vi "主界面Z140.vi"() -> ()   [LabVIEW 2013]
uses:
  TCP/S7Ref.vi
panel:
  in  "复位":bool
  out "通讯状态":bool
  out "上序不合格":bool
  out "上序合格":bool
  out "本序不合格":bool
  out "本序合格":bool
  in  "停止":bool
  out "自动工步号":i32
  out "芯片ID":string
  out "压装工位操作状态":string
  in  "联线按钮":bool
  in  "选项卡控件":enum32{"自动界面", "手动界面", "参数"}(tab)
  out "胶塞在位":bool
  out "该型号检验辅具全在位，可以开始检验":bool
  out "辅具10":bool
  out "辅具9":bool
  out "辅具5":bool
  out "辅具4":bool
  out "辅具3":bool
  out "辅具2":bool
  out "辅具1":bool
  out "辅具6":bool
  in  "气缸进":bool
  in  "气缸退":bool
  out "联线状态":bool
  out "气压报警":bool
  in  "手动操作":bool
  in  "簇":T1
  out "员工ID":string
  out "员工姓名":string
  in  "型号选择":u16(ring)=1 items=["J709", "J706"]
  in  "参数加载":bool
  in  "产品ID":string
  # "芜湖机械转向器装配线"
  # "出厂检验台"
  # "Q14070机械转向器装配线"
  # "湖北唯思凌科装备制造有限公司 设计开发 (C)2015"
  # "检验前请检查辅具是否在位"
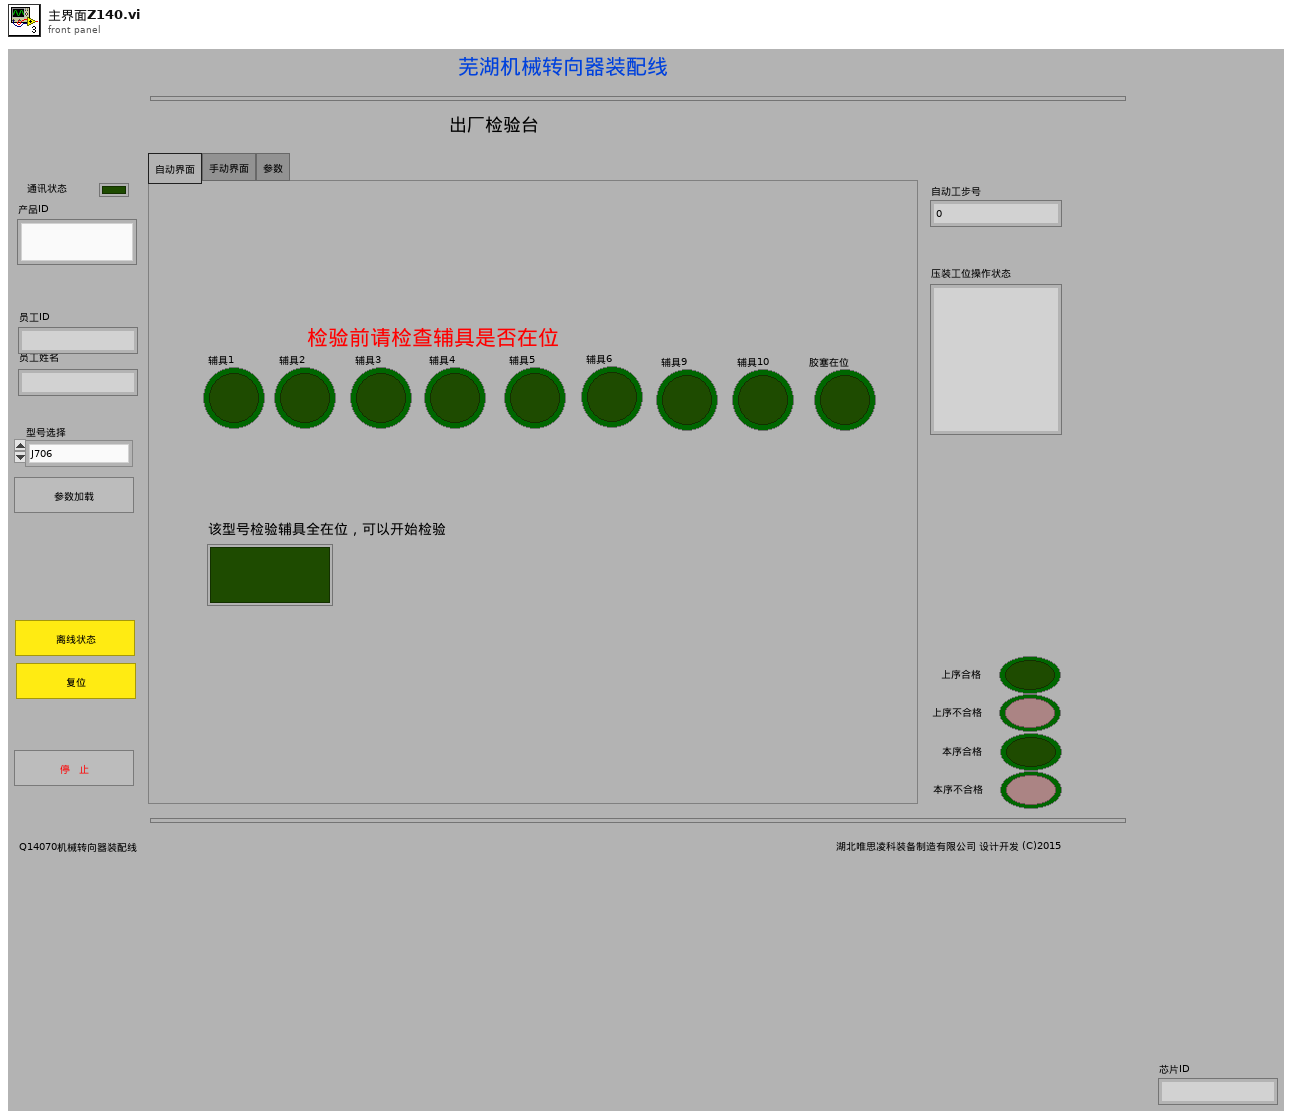
[diagram p1: front panel]
types:
  T1 = cluster{"布尔":bool, "布尔 2":bool, "布尔 3":bool, "布尔 4":bool, "布尔 5":bool, "布尔 6":bool, "布尔 7":bool, "布尔 8":bool, "布尔 9":bool}
  T2 = enum32{"Invalid", "Standard", "Closed", "Hidden", "Minimized", "Maximized"}
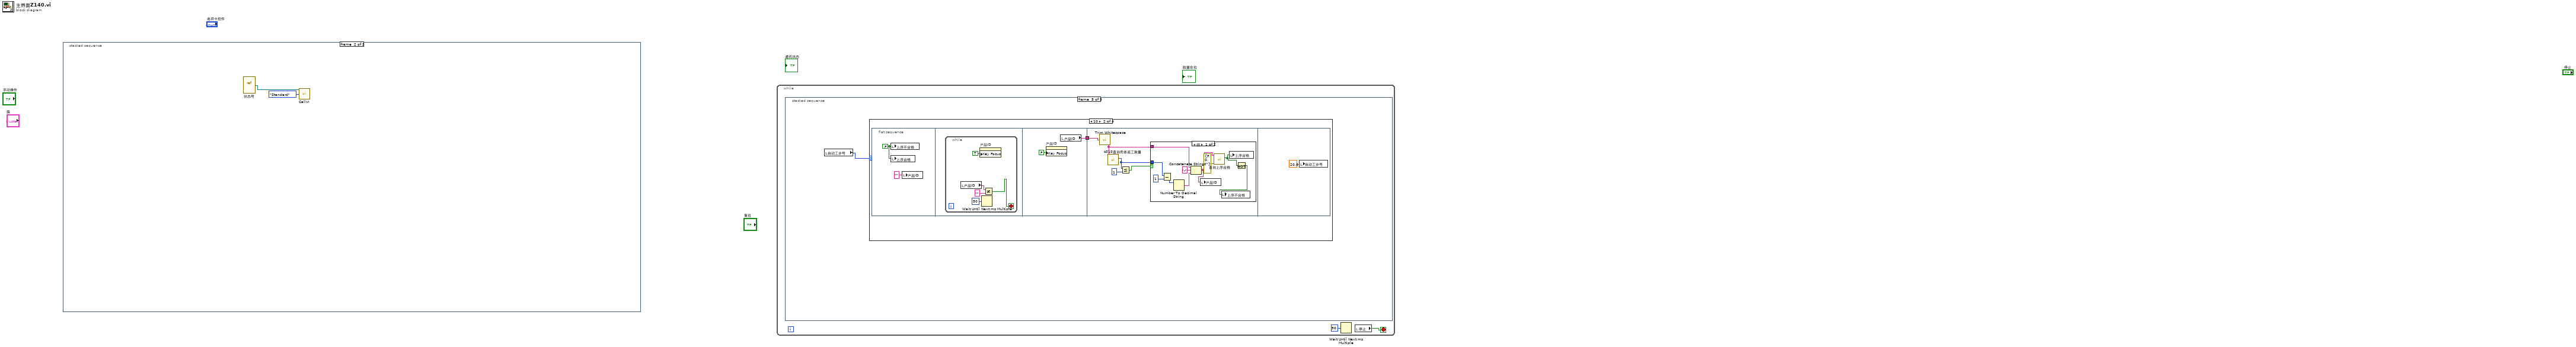
[diagram p0: block diagram]
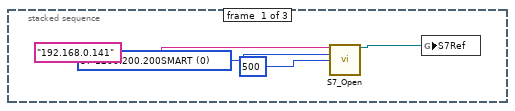
[diagram p2: hidden frame]
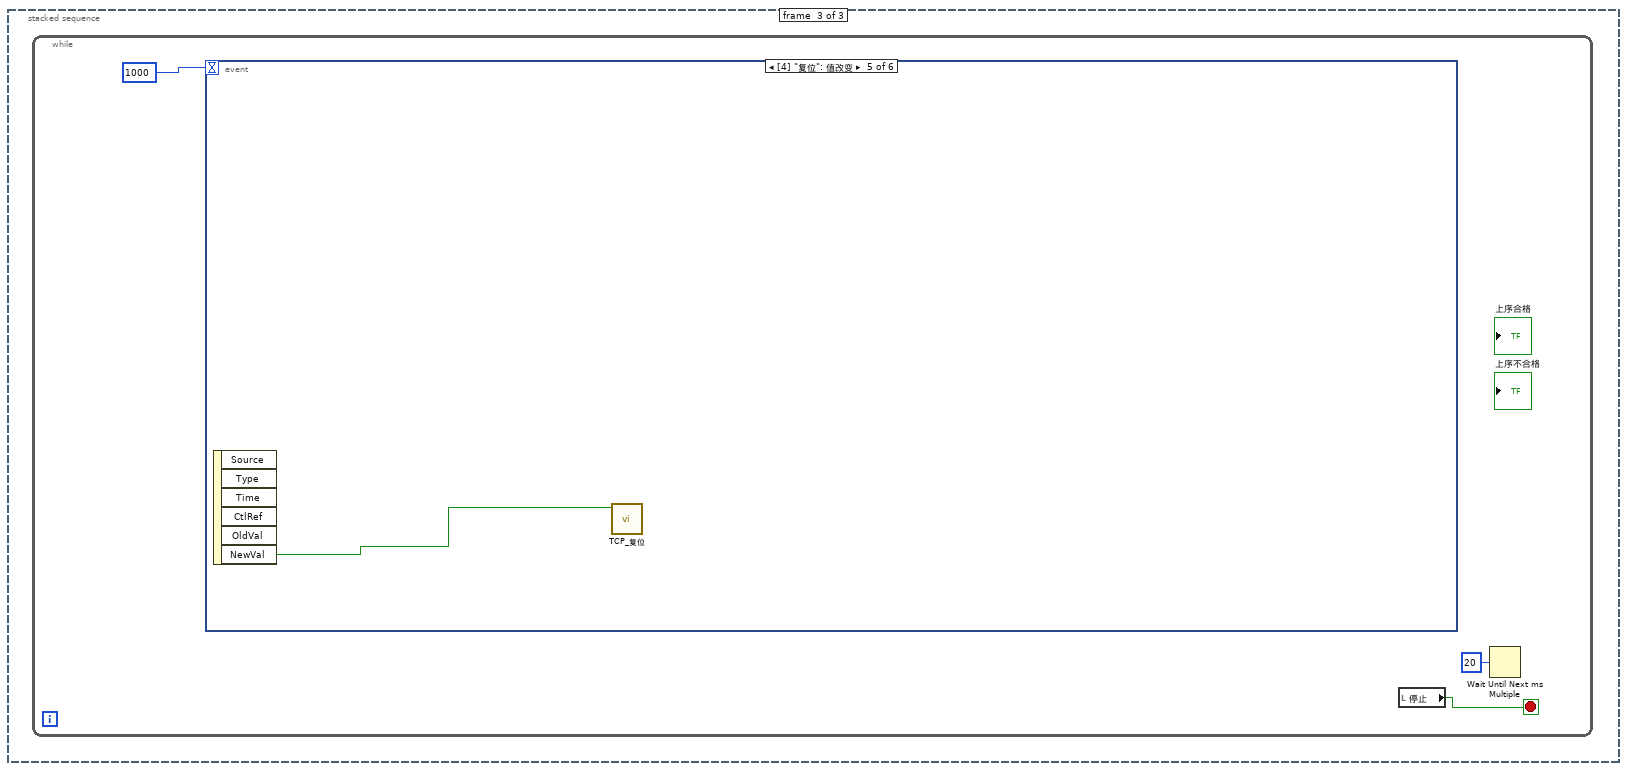
[diagram p3: hidden frame]
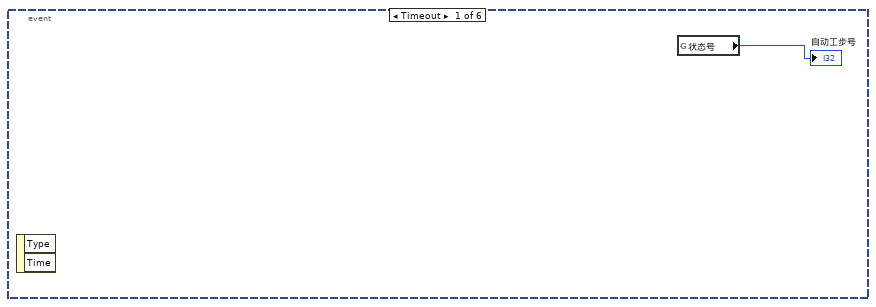
[diagram p4: hidden frame]
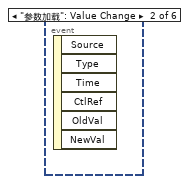
[diagram p5: hidden frame]
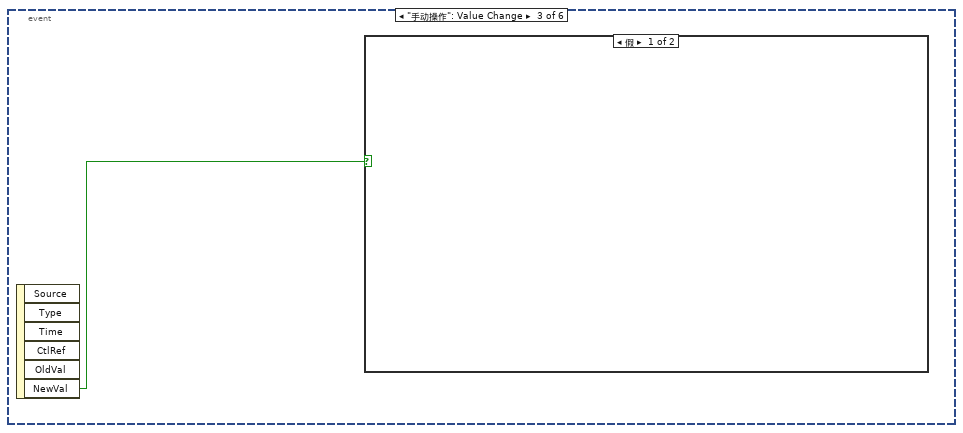
[diagram p6: hidden frame]
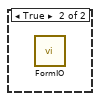
[diagram p7: hidden frame]
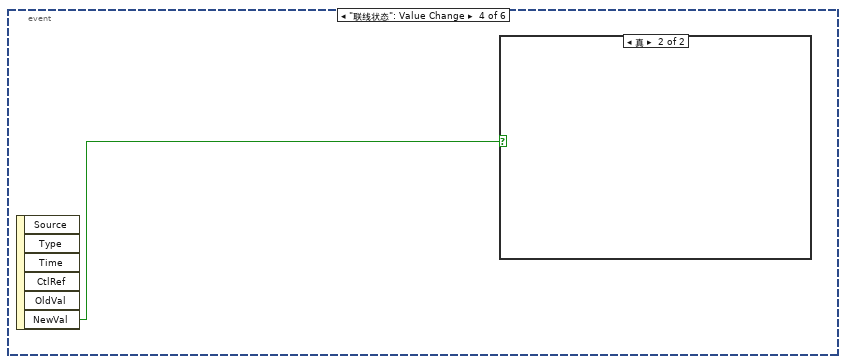
[diagram p8: hidden frame]
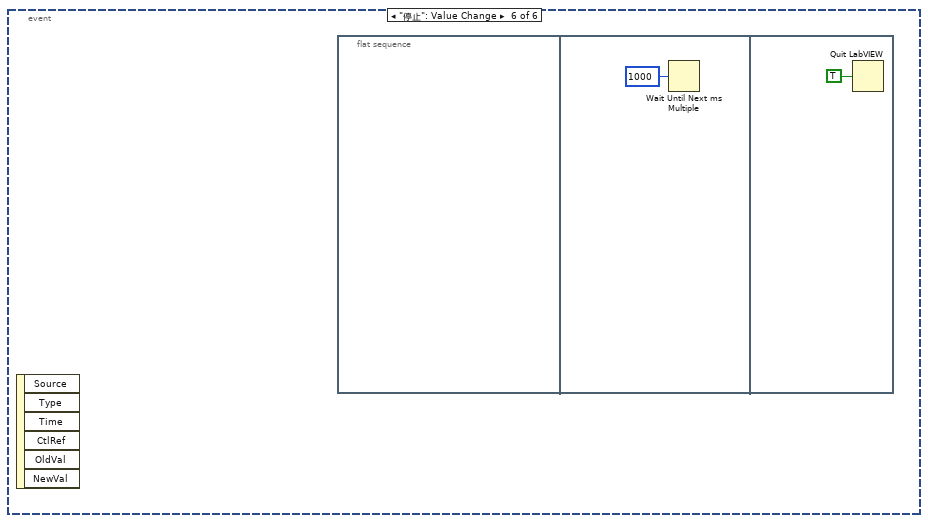
[diagram p10: hidden frame]
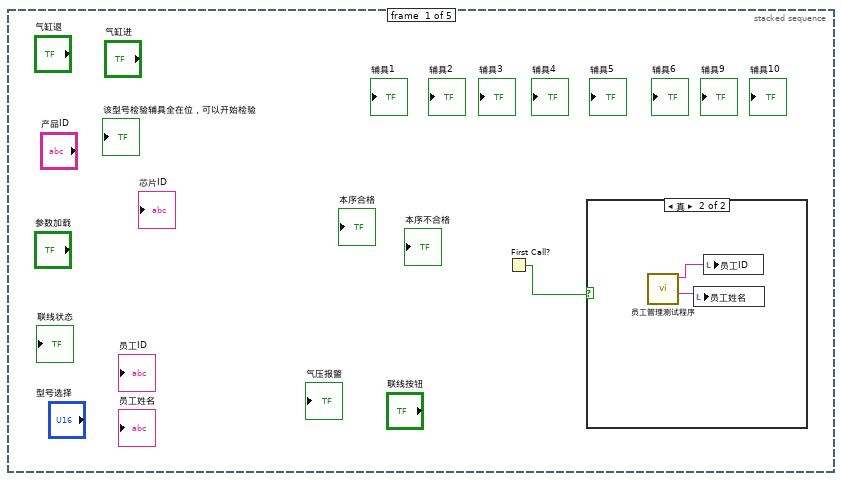
[diagram p11: hidden frame]
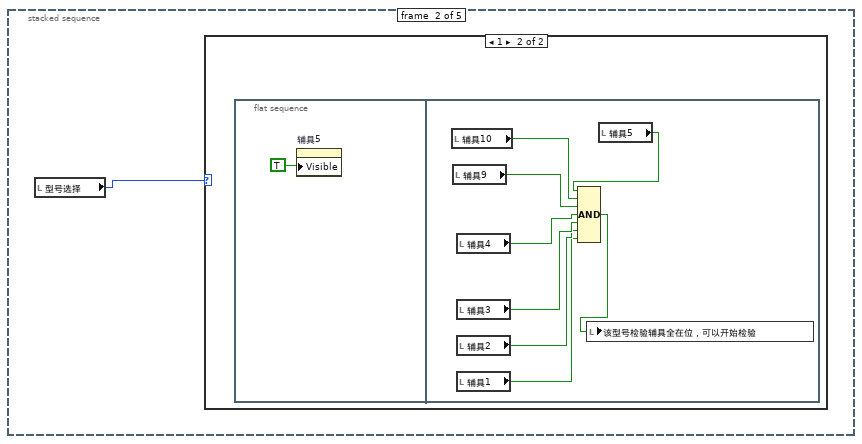
[diagram p13: hidden frame]
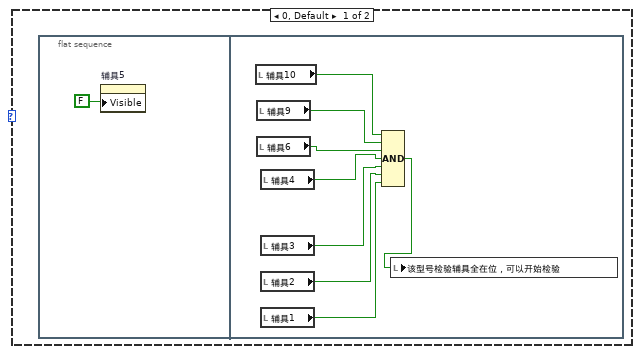
[diagram p14: hidden frame]
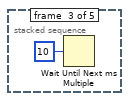
[diagram p15: hidden frame]
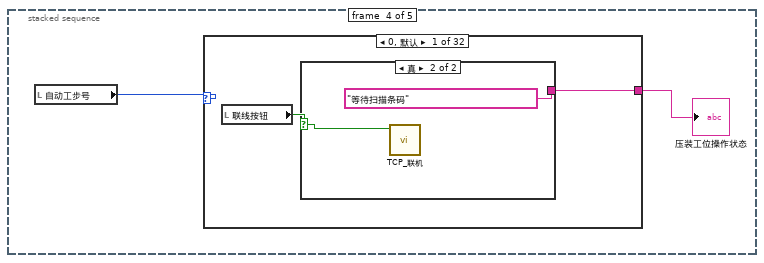
[diagram p16: hidden frame]
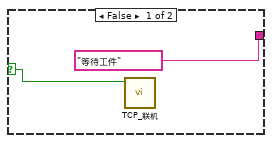
[diagram p17: hidden frame]
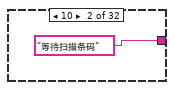
[diagram p18: hidden frame]
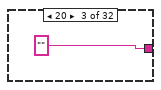
[diagram p19: hidden frame]
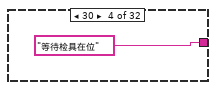
[diagram p20: hidden frame]
diagram:
  n1 = stacked-sequence {
    frame #0 {
      w3 = u8 0 items=["S7-1200.200.200SMART"=0, "S7-300"=2, "S7-400"=3] ("PLC 系列")
      n2 = call "S7_Open .vi"("IP 地址"="192.168.0.141", "PLC 系列"=w3, "超时（MS）"=500) -> ("TCP"=w1:refnum<k5>)  [unwired: 9 in, 3 out]
      n3 = global write "S7Ref.vi" "S7Ref"(w1) -> ()
    }
    frame #1 {
      n4 = vi-ref "状态号.vi"() -> (w6:refnum<vi>)
      n5 = call "CallVI.vi"("VI引用"=w6, "状态"=T2."Standard") -> ()  [unwired: 12 in, 2 out]
    }
    frame #2 {
      n6 = while {
        stop <- w7 stop-if-true
        n7 = event shown="[4] \"复位\": 值改变" {
          selector: _ -> [_ _ _ _ _ _]
          dyn-events: _ -> [_ _ _ _ _ _]
          timeout: 1000 -> [_ _ _ _ _ _]
          event Timeout {
            n8 = event-data() -> ()  [unwired: 3 out]
            n9 = global read "全局 1.vi" "状态号"() -> (→"自动工步号":i32)
          }
          event "参数加载": Value Change {
            n10 = event-data() -> ()  [unwired: 7 out]
          }
          event "手动操作": Value Change {
            n11 = event-data() -> ("NewVal"=w11:bool)  [unwired: 6 out]
            n12 = case shown="假" w11 {
              frame False {
              }
              frame True {
                n13 = call "FormIO.vi"() -> ()  [unwired: 12 in]
              }
            }
          }
          event "联线状态": Value Change {
            n14 = event-data() -> ("NewVal"=w12:bool)  [unwired: 6 out]
            n15 = case shown="真" w12 {
              frame False {
              }
              frame True {
              }
            }
          }
          event "复位": Value Change {
            n16 = event-data() -> ("NewVal"=w13:bool)  [unwired: 6 out]
            n17 = call "TCP_复位.vi"("联机"=w13) -> ()  [unwired: 11 in]
          }
          event "停止": Value Change {
            n18 = event-data() -> ()  [unwired: 7 out]
            n19 = flat-sequence {
              frame #0 {
              }
              frame #1 {
                n20 = Wait Until Next ms Multiple(millisecond multiple=u32 1000 ("毫秒倍数")) -> ()  [unwired: 1 out]
              }
              frame #2 {
                n21 = Quit LabVIEW(quit? (T)=TRUE ("停止？(T)")) -> ()
              }
            }
          }
        }
        n22 = local read "停止"() -> (w7:bool)
        n23 = Wait Until Next ms Multiple(millisecond multiple=u32 20 ("毫秒倍数")) -> ()  [unwired: 1 out]
      }
    }
  }
  n24 = while {
    stop <- w16 stop-if-true
    n25 = stacked-sequence {
      frame #0 {
        n26 = First Call?() -> (First Call?: T/F=w18:bool)
        n27 = case shown="真" w18 {
          frame False {
          }
          frame True {
            n28 = call "员工管理测试程序.vi"() -> ("员工姓名"=w20:string, "员工ID"=w19:string)  [unwired: 10 in]
            n29 = local write "员工姓名"(w20) -> ()
            n30 = local write "员工ID"(w19) -> ()
          }
        }
      }
      frame #1 {
        n31 = local read "型号选择"() -> (w21:u16)
        n32 = case shown="1" w21 {
          frame 0, Default {
            n33 = flat-sequence {
              frame #0 {
                n34 = property on="辅具5" class="Bool (严格)"("Visible"=FALSE ("可见")) -> ()  [unwired: 2 in, 2 out]
              }
              frame #1 {
                n35 = local read "辅具10"() -> (w30:bool)
                n36 = local read "辅具9"() -> (w29:bool)
                n37 = local read "辅具6"() -> (w28:bool)
                n38 = local read "辅具4"() -> (w27:bool)
                n39 = local read "辅具3"() -> (w26:bool)
                n40 = local read "辅具2"() -> (w25:bool)
                n41 = local read "辅具1"() -> (w24:bool)
                n42 = Compound Arithmetic op=AND(w30, w29, w28, w27, w26, w25, w24) -> (w23:bool)
                n43 = local write "该型号检验辅具全在位，可以开始检验"(w23) -> ()
              }
            }
          }
          frame 1 {
            n44 = flat-sequence {
              frame #0 {
                n45 = property on="辅具5" class="Bool (严格)"("Visible"=TRUE ("可见")) -> ()  [unwired: 2 in, 2 out]
              }
              frame #1 {
                n46 = local read "辅具10"() -> (w39:bool)
                n47 = local read "辅具9"() -> (w38:bool)
                n48 = local read "辅具4"() -> (w37:bool)
                n49 = local read "辅具3"() -> (w36:bool)
                n50 = local read "辅具2"() -> (w35:bool)
                n51 = local read "辅具1"() -> (w34:bool)
                n52 = local read "辅具5"() -> (w32:bool)
                n53 = Compound Arithmetic op=AND(w32, w39, w38, w37, w36, w35, w34) -> (w33:bool)
                n54 = local write "该型号检验辅具全在位，可以开始检验"(w33) -> ()
              }
            }
          }
        }
      }
      frame #2 {
        n55 = Wait Until Next ms Multiple(millisecond multiple=u32 10 ("毫秒倍数")) -> ()  [unwired: 1 out]
      }
      frame #3 {
        n56 = local read "自动工步号"() -> (w42:i32)
        n57 = case shown="0, 默认" w42 {
          tunnel: [w44 "等待扫描条码" ("工步操作状态") "" ("工步操作状态") "等待检具在位" ("工步操作状态") "左右拉杆检测在位" ("工步操作状态") "按启动按钮" ("工步操作状态") "检拉杆在位" ("工步操作状态") "拉杆不在位，请将拉杆安装到位" ("工步操作状态") "按启动按钮" ("工步操作状态") "气缸前进" ("工步操作状态") "检胶塞在位" ("工步操作状态") "请取螺纹环规M12*1.5（通）" ("工步操作状态") "取料错误，请放回，并重新取料轴承B" ("工步操作状态") "请放螺纹环规M12*1.5（通）" ("工步操作状态") "请取螺纹环规M12*1.5（止）" ("工步操作状态") "压装过程中碰到光幕，请按启动按钮，气缸返回，重新进行压装\n" ("工步操作状态") "请放回螺纹环规M12*1.5（止）" ("工步操作状态") " 请取球销内六角扳手" ("工步操作状态") " 请放回球销内六角扳手" ("工步操作状态") " 请取花键规（通）" ("工步操作状态") "请放回花键规（通）" ("工步操作状态") "请取花键规（止）" ("工步操作状态") "请放回花键规（止）" ("工步操作状态") "请取螺纹塞规M6" ("工步操作状态") "请放回螺纹塞规M6" ("工步操作状态") "请取M14叉扳手" ("工步操作状态") "请放回M14叉扳手" ("工步操作状态") "" ("工步操作状态") "气缸退回" ("工步操作状态") "胶塞漏装，请复位" ("工步操作状态") "压装不合格" ("工步操作状态") "数据上传完成" ("工步操作状态")] -> w41
          frame 0, Default {
            n58 = local read "联线按钮"() -> (w43:bool)
            n59 = case shown="真" w43 {
              selector: w43 -> [w45 w47]
              tunnel: ["等待工件" ("工步操作状态") "等待扫描条码" ("工步操作状态")] -> w44
              frame False {
                n60 = call "TCP_联机.vi"("联机"=w45) -> ()  [unwired: 11 in]
              }
              frame True {
                n61 = call "TCP_联机.vi"("联机"=w47) -> ()  [unwired: 11 in]
              }
            }
          }
          frame 10 {
          }
          frame 20 {
          }
          frame 30 {
          }
          frame 31 {
          }
          frame 32 {
          }
          frame 35 {
          }
          frame 38 {
          }
          frame 40 {
          }
          frame 45 {
          }
          frame 47 {
          }
          frame 50 {
          }
          frame 51 {
          }
          frame 60 {
          }
          frame 70 {
          }
          frame 71 {
          }
          frame 80 {
          }
          frame 90 {
          }
          frame 100 {
          }
          frame 110 {
          }
          frame 120 {
          }
          frame 130 {
          }
          frame 140 {
          }
          frame 150 {
          }
          frame 160 {
          }
          frame 170 {
          }
          frame 180 {
          }
          frame 190 {
          }
          frame 200 {
          }
          frame 700 {
          }
          frame 800 {
          }
          frame 900 {
          }
        }
        "压装工位操作状态" <- w41
      }
      frame #4 {
        n62 = local read "自动工步号"() -> (w80:i32)
        n63 = case shown="10" w80 {
          frame 0, Default {
          }
          frame 10 {
            n64 = flat-sequence {
              tunnel: [w89] -> w81
              tunnel: w81 -> [w95]
              frame #0 {
                w83 = FALSE ("上序不合格")
                n65 = local write "上序不合格"(w83) -> ()
                n66 = local write "上序合格"(w83) -> ()
                n67 = local write "产品ID"("" ("产品ID")) -> ()
              }
              frame #1 {
                n68 = while {
                  stop <- w84 stop-if-true
                  n69 = local read "产品ID"() -> (w88:string)
                  n70 = property on="产品ID" class="Str"("Key Focus"=TRUE ("键选中")) -> ()  [unwired: 2 in, 2 out]
                  n71 = Wait Until Next ms Multiple(millisecond multiple=u32 50 ("毫秒倍数")) -> ()  [unwired: 1 out]
                  n72 = Not Equal?(x=w88, y="") -> (x != y?=w84:bool)
                }
              }
              frame #2 {
                n73 = property on="产品ID" class="Str"("Key Focus"=FALSE ("键选中")) -> ()  [unwired: 2 in, 2 out]
                n74 = local read "产品ID"() -> (w89:string)
              }
              frame #3 {
                n75 = call <vilib>:"Trim Whitespace.vi"("string"=w95) -> ("trimmed string"=w92:string)  [unwired: 1 in]
                n76 = call "z010查询壳体返工数量.vi"("转向器总成ID"=w92) -> ("Rows Fetched"=w91:i32)  [unwired: 8 in, 2 out]
                n77 = Less Or Equal?(x=w91, y=1) -> (x <= y?=w93:bool)
                n78 = case shown="假" w93 {
                  tunnel: w92 -> [w100 w106]
                  tunnel: w91 -> [w105 _]
                  frame False {
                    n79 = Subtract(x=w105, y=1) -> (x-y=w103:i32)
                    n80 = Number To Decimal String(number=w103) -> (decimal integer string=w102:string)  [unwired: 1 in]
                    n81 = Concatenate Strings(w100, "-" ("字符串"), w102) -> (w96:string)
                    n82 = local write "产品ID"(w96) -> ()
                    n83 = call "查询上序合格.vi"("error in (no error)"=errorcluster {"status"=FALSE, "code"=0, "source"=""}, "产品ID"=w96) -> ("上序合格"=w98:bool)  [unwired: 7 in, 2 out]
                    n84 = local write "上序合格"(w98) -> ()
                    n85 = Not(x=w98) -> (.not. x?=w97:bool)
                    n86 = local write "上序不合格"(w97) -> ()
                  }
                  frame True {
                    n87 = call "查询上序合格.vi"("error in (no error)"=errorcluster {"status"=FALSE, "code"=0, "source"=""}, "产品ID"=w106) -> ("上序合格"=w108:bool)  [unwired: 7 in, 2 out]
                    n88 = local write "上序合格"(w108) -> ()
                    n89 = Not(x=w108) -> (.not. x?=w107:bool)
                    n90 = local write "上序不合格"(w107) -> ()
                  }
                }
              }
              frame #4 {
                n91 = local write "自动工步号"(20.0 ("自动工步号")) -> ()
              }
            }
          }
          frame 600 {
            n92 = flat-sequence {
              frame #0 {
                n93 = local read "产品ID"() -> (w111:string)
                n94 = local read "员工姓名"() -> (w115:string)
                n95 = Build Array(w111, w115, "1" ("元素"), "1" ("元素")) -> (w112:string[])
                n96 = call "数据库更新.vi"("设备号"="14", "数据"=w112) -> ()  [unwired: 13 in, 1 out]
              }
              frame #1 {
                n97 = local write "产品ID"("" ("产品ID")) -> ()
                n98 = local write "自动工步号"(610.0 ("自动工步号")) -> ()
              }
            }
          }
          frame 610 {
            w120 = FALSE ("上序不合格")
            n99 = local write "上序不合格"(w120) -> ()
            n100 = local write "上序合格"(w120) -> ()
            n101 = local write "产品ID"("" ("产品ID")) -> ()
            n102 = Wait (ms)(milliseconds to wait=u32 50 ("等待时间（毫秒）")) -> ()  [unwired: 1 out]
          }
        }
      }
    }
    n103 = Wait Until Next ms Multiple(millisecond multiple=u32 50 ("毫秒倍数")) -> ()  [unwired: 1 out]
    n104 = local read "停止"() -> (w16:bool)
  }
